vi "HAM Digital Radio - UI.vi"(8 "error in (no error)":errorcluster, 11 "Queues":T1) -> (0 "error out":errorcluster)   [LabVIEW 2013]
uses:
  STYPS/HDR - Queues.ctl
panel:
  in  "settings":bool
  in  "clear":bool
  in  "chat_user":string
  in  "send":bool
  in  "chat_send":string
  out "chat_main":string
  out "DATA str":string
  out "STOP":bool
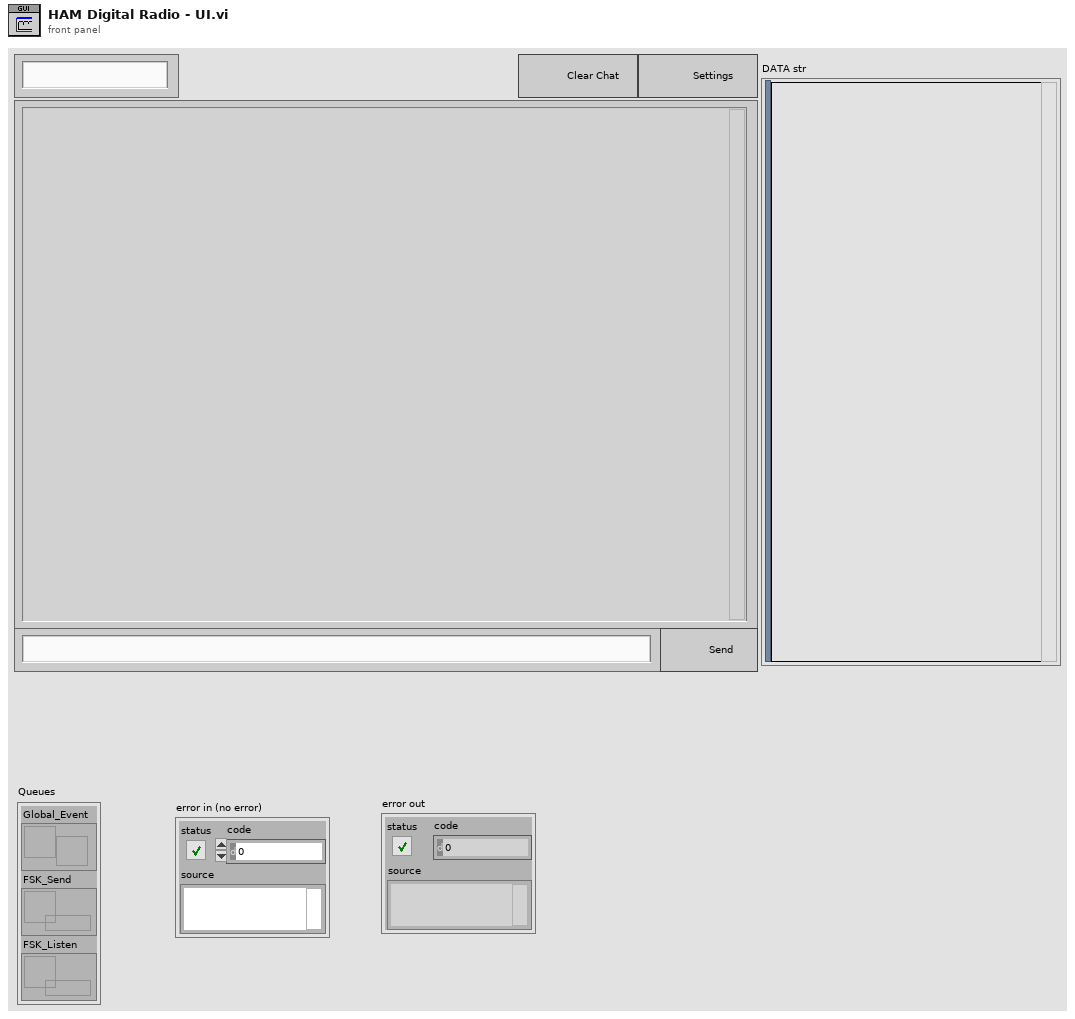
[diagram p1: front panel]
types:
  T1 = typedef "HDR - Queues.ctl" = cluster{"Global_Event":refnum<user-event>, "FSK_Send":refnum<queue>, "FSK_Listen":refnum<queue>}
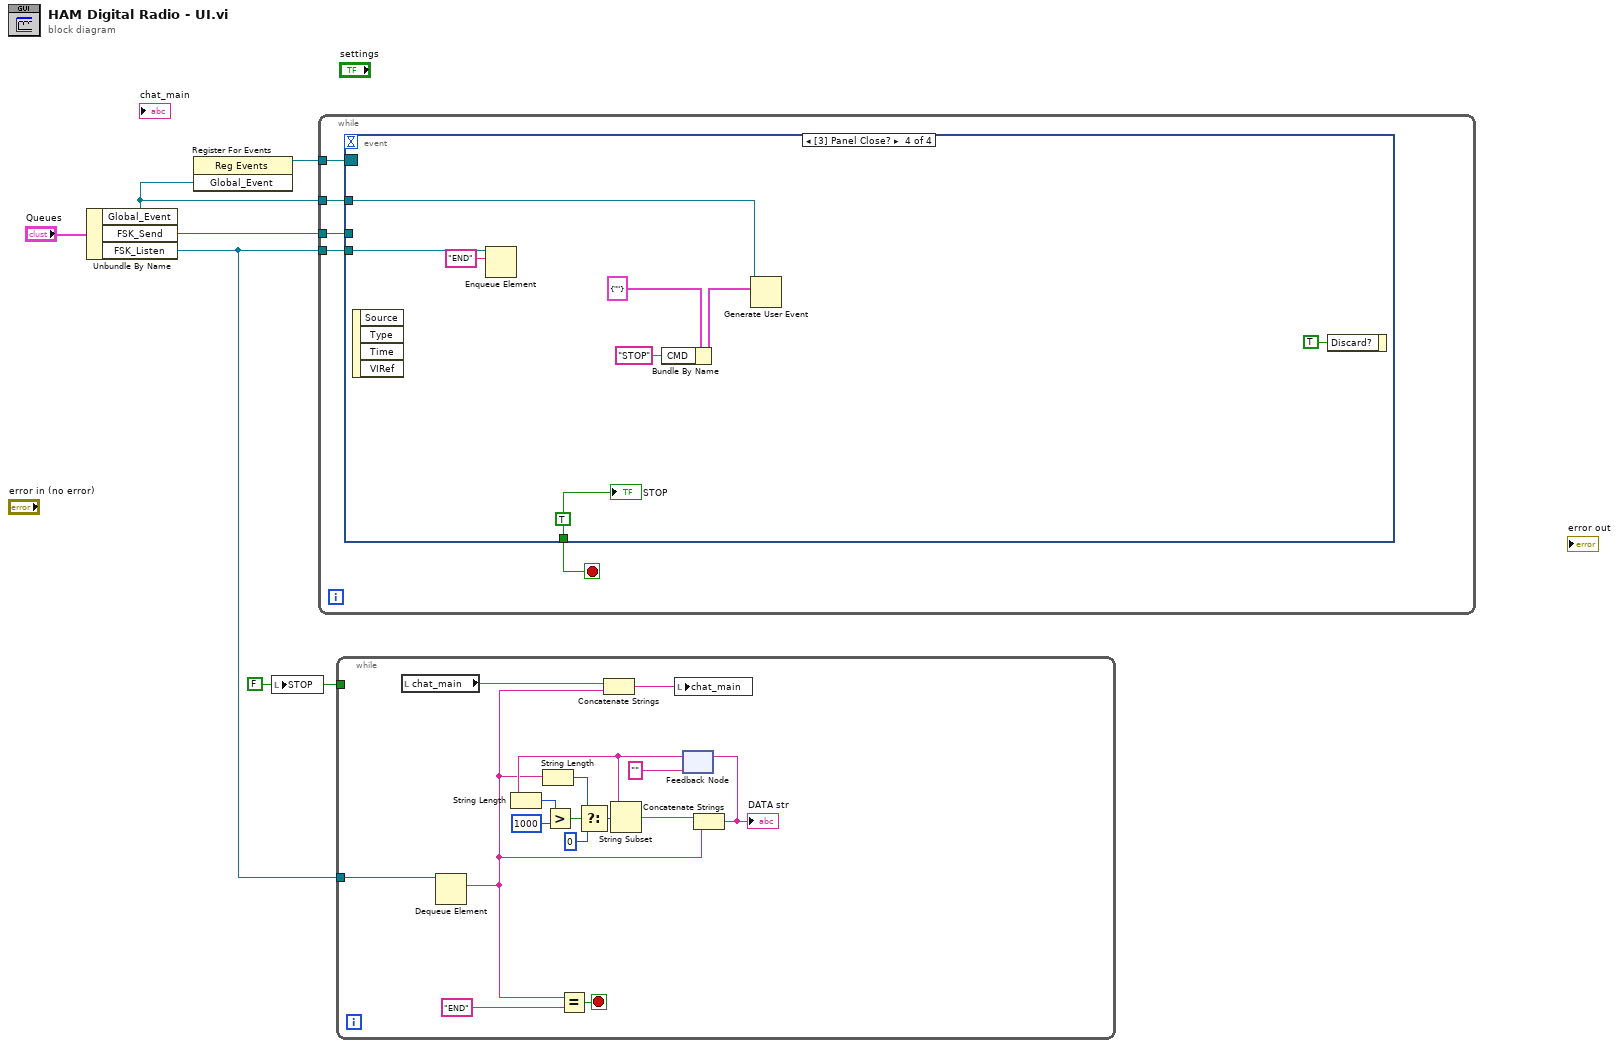
[diagram p0: block diagram]
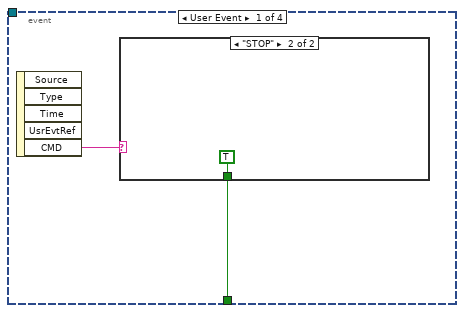
[diagram p2: hidden frame]
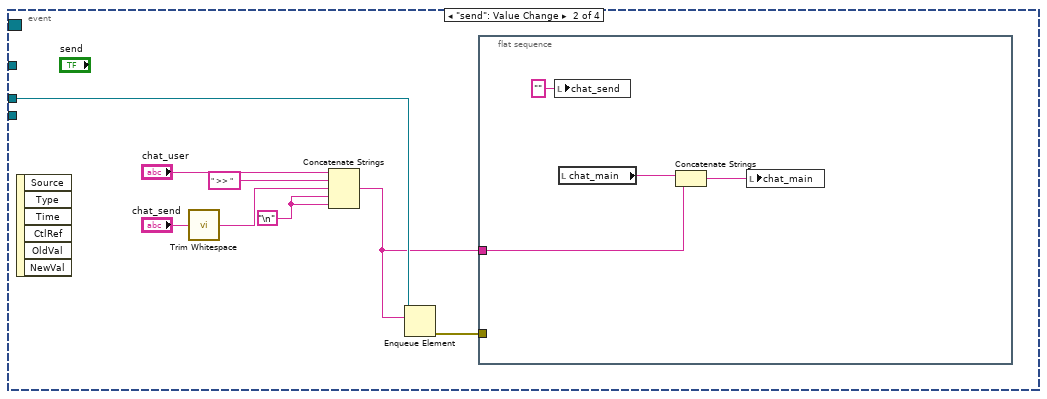
[diagram p4: hidden frame]
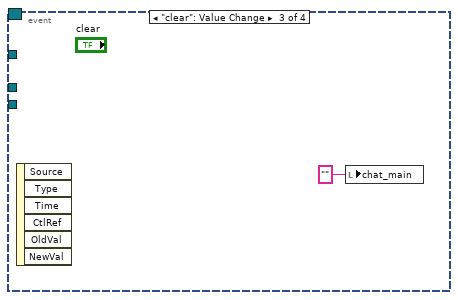
[diagram p5: hidden frame]
diagram:
  w1 = FALSE ("STOP")
  n1 = Unbundle By Name("Queues") -> ("Global_Event"=w3:refnum<user-event>, "FSK_Send"=w4:refnum<queue>, "FSK_Listen"=w2:refnum<queue>)
  n2 = register-events(w3) -> (reference out=w6:refnum<event-registration>)  [unwired: 2 in, 1 out]
  n3 = local write "STOP"(w1) -> ()
  n4 = while {
    tunnel: w6 -> [w11]
    tunnel: w4 -> [w9]
    tunnel: w3 -> [w8]
    tunnel: w2 -> [w7]
    stop <- w10 stop-if-true
    n5 = event shown="[3] Panel Close?" {
      selector: w11 -> [_ _ _ _]
      dyn-events: _ -> [_ _ _ _]
      timeout: _ -> [_ _ _ _]
      tunnel: [w12 _ _ w28] -> w10
      tunnel: w9 -> [_ w18 _ _]
      tunnel: w8 -> [_ _ _ w34]
      tunnel: w7 -> [_ _ _ w30]
      event User Event {
        n6 = event-data() -> ("CMD"=w13:string)  [unwired: 1 in, 4 out]
        n7 = case shown="\"STOP\"" w13 {
          tunnel: [_ TRUE] -> w12
          frame Default {
          }
          frame "STOP" {
          }
        }
      }
      event "send": Value Change {
        w15 = "\n"
        n8 = event-data() -> ()  [unwired: 1 in, 6 out]
        n9 = call <vilib>:"Trim Whitespace.vi"("string"="chat_send") -> ("trimmed string"=w19:string)  [unwired: 1 in]
        n10 = Concatenate Strings("chat_user", " >> " ("string"), w19, w15, w15) -> (w16:string)
        n11 = Enqueue Element(queue=w18, element=w16) -> (error out=w17:errorcluster)  [unwired: 2 in, 2 out]
        n12 = flat-sequence {
          tunnel: w17 -> [_]
          tunnel: w16 -> [w24]
          frame #0 {
            n13 = local write "chat_send"("" ("chat_send")) -> ()
            n14 = local read "chat_main"() -> (w25:string)
            n15 = Concatenate Strings(w25, w24) -> (w23:string)
            n16 = local write "chat_main"(w23) -> ()
          }
        }
      }
      event "clear": Value Change {
        n17 = event-data() -> ()  [unwired: 1 in, 6 out]
        n18 = local write "chat_main"("" ("chat_main")) -> ()
      }
      event Panel Close? {
        w28 = TRUE
        n19 = event-data() -> ()  [unwired: 1 in, 4 out]
        n20 = Enqueue Element(queue=w30, element="END") -> ()  [unwired: 2 in, 3 out]
        n21 = Bundle By Name(cluster=cluster{"CMD":string} {"CMD"=""} ("event data"), "CMD"="STOP") -> (w32:cluster{"CMD":string})
        n22 = Generate User Event(user event=w34, event data cluster=w32) -> ()  [unwired: 2 in, 2 out]
        n23 = event-data("Discard?"=TRUE) -> ()  [unwired: 1 in, 1 out]
        "STOP" <- w28
      }
    }
  }
  n24 = while {
    tunnel: w2 -> [w51]
    tunnel: w1 -> [_]
    stop <- w36 stop-if-true
    n25 = local read "chat_main"() -> (w39:string)
    n26 = Dequeue Element(queue=w51) -> (element=w38:string)  [unwired: 2 in, 3 out]
    n27 = String Length(string=w38) -> (length=w45:i32)
    n28 = Equal?(x=w38, y="END") -> (x = y?=w36:bool)
    n29 = Concatenate Strings(w39, w38) -> (w40:string)
    n30 = local write "chat_main"(w40) -> ()
    n31 = feedback #1("" ("*(type *) &x")) -> (w49:string)
    n32 = String Length(string=w49) -> (length=w41:i32)
    n33 = Greater?(x=w41, y=1000) -> (0:w43:bool)
    n34 = Select(t=w45, s=w43, f=0) -> (s? t:f=w47:i32)
    n35 = String Subset(string=w49, offset (0)=w47) -> (substring=w48:string)  [unwired: 1 in]
    n36 = Concatenate Strings(w48, w38) -> (w50:string)
    "DATA str" <- w50
    n37 = feedback-in #1(w50) -> ()
  }
